vi "KlingerV2 OriginSearch.vi"(0 "VISA Rsrc":refnum<visa-resource-name>="SR530", 1 "UnitDem":u8(ring)=2 caption="Unités\nDemandées" items=["Pas", "mm", "ps"], 5 "Axe":u8(ring) items=["W", "X", "Y", "Z"], 7 "Moving Ref":refnum<vi>, 9 "Position Ref":refnum<vi>, 11 "error in":errorcluster, 12 "Set as Zero":bool) -> (2 "Pos Init":dbl caption="Position Initiale", 3 "Moving":bool caption="Déplacement\nen cours", 4 "PLimit":bool caption="Limite +", 6 "NLimit":bool caption="Limite -", 10 "Position":dbl format="%#.1f", 14 "Indcomm":string caption="Indicateur de commande", 15 "error out":errorcluster)   [LabVIEW 2019]
doc: "Ce VI envoie une commande de Mise à 0 au controlleur Klinger MC4. \n\nAxe : Sélectionner l'axe sur lequel effectuer la mise à zéro\n\nMoving Ref : Connecter une référence permet l'actualisation d'un afficheur de déplacement en cours en temp réelle\n\nPosition Ref: Connecter une référence permet l'actualisation d'un afficheur de position actuelle en temp réelle\n\nLimite + : Indique l'atteinte de l'interrupeur de fin de course positif\n\nLimite - : Indique l'atteinte de l'interrupeur de fin de course négatif\n\nPosition: Indique la position finale"
panel:
  out "Message D'erreur":string
  out "Erreur":bool
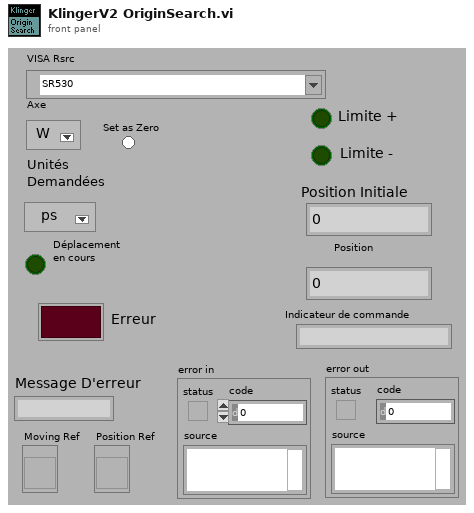
[diagram p1: front panel]
types:
  T1 = enum16{"Dem Pos Init", "Lire Pos Init", "Envoie Comm", "Dem Statut", "Lire Statut", "Attend RQS", "Erreur GPIB", "Dépl incomp", "Dépl comp"}
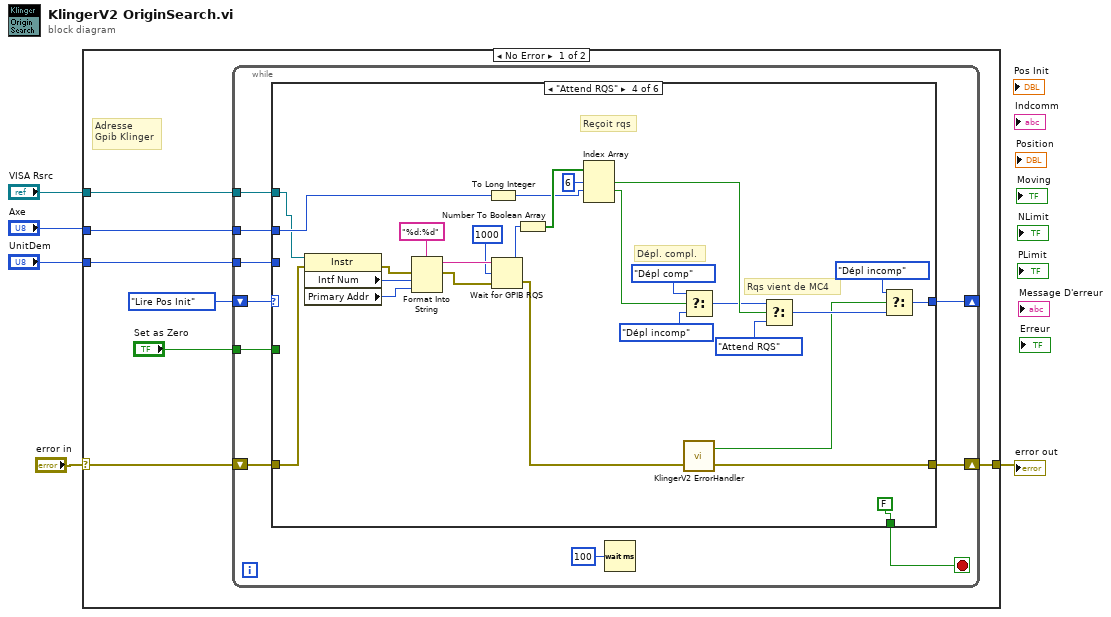
[diagram p0: block diagram]
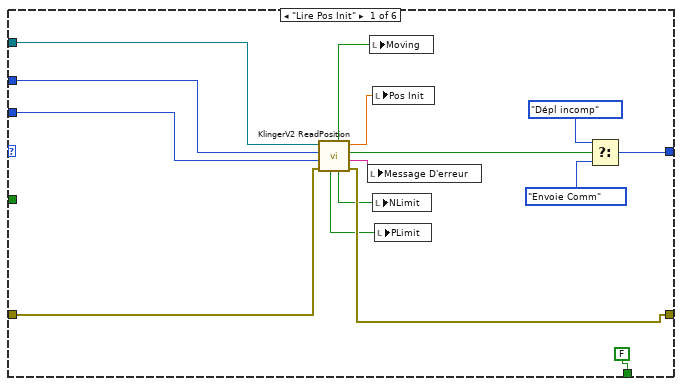
[diagram p2: hidden frame]
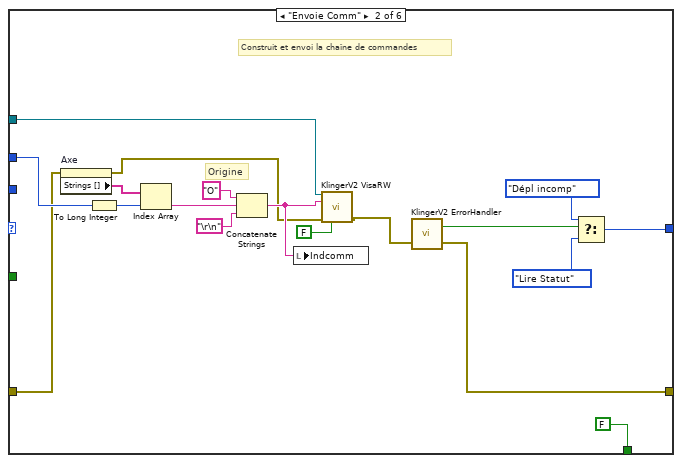
[diagram p3: hidden frame]
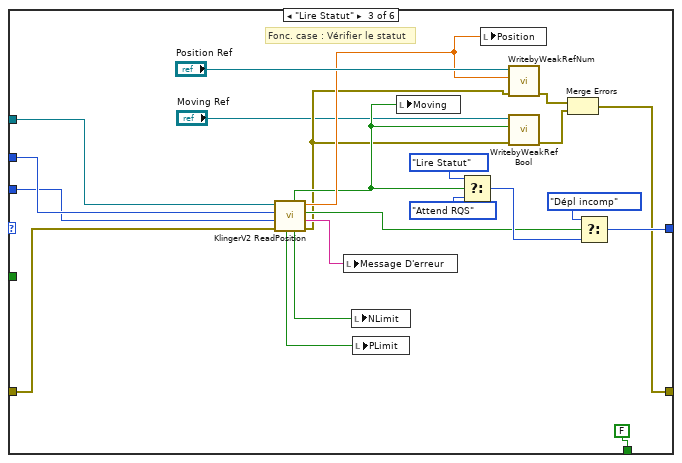
[diagram p4: hidden frame]
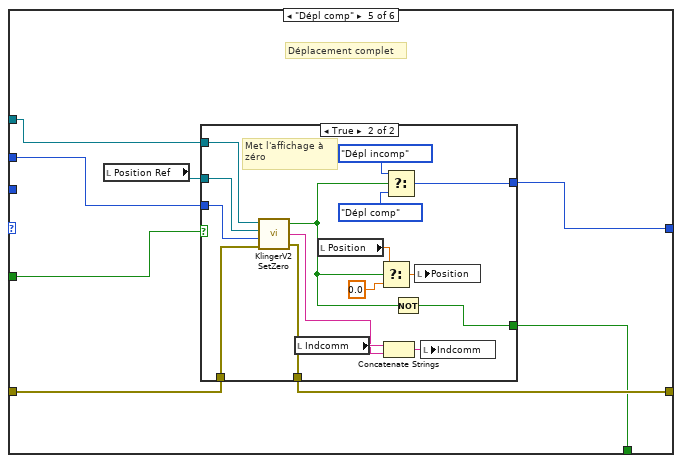
[diagram p5: hidden frame]
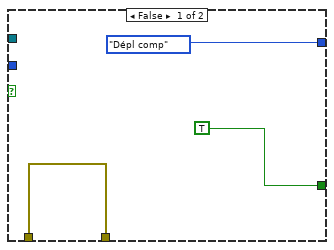
[diagram p6: hidden frame]
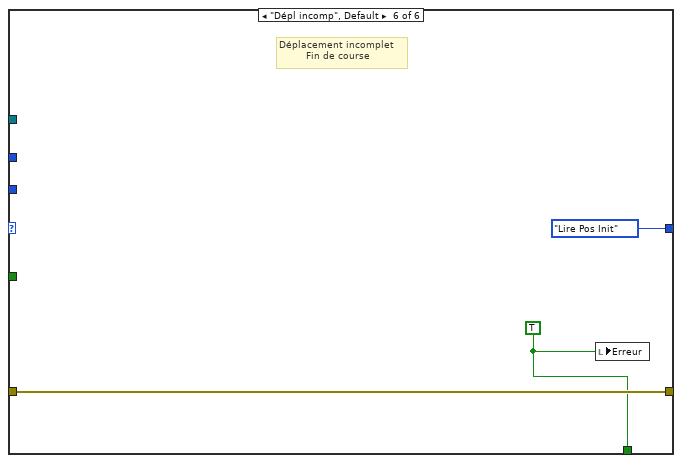
[diagram p7: hidden frame]
diagram:
  n1 = case shown="No Error" "error in" {
    selector: "error in" -> [w11 w135]
    tunnel: [w12 w135] -> w5
    tunnel: "VISA Rsrc" -> [w8 _]
    tunnel: "UnitDem" -> [w7 _]
    tunnel: "Axe" -> [w6 _]
    frame No Error {
      # "Adresse \nGpib Klinger"
      n2 = while {
        shift-right: [w21] -> w12
        shift-left: w11 -> [w20]
        tunnel: w6 -> [w19]
        shift-right: [w16] -> _
        shift-left: T1."Lire Pos Init" ("f") -> [w17]
        tunnel: "Set as Zero" -> [w15]
        tunnel: w7 -> [w14]
        tunnel: w8 -> [w13]
        stop <- w22 stop-if-true
        n3 = case shown="\"Attend RQS\"" w17 {
          tunnel: [FALSE FALSE FALSE FALSE w107 w132] -> w22
          tunnel: [w33 w45 w58 w90 w109 w133] -> w21
          tunnel: w20 -> [w31 w39 w71 w80 w110 w133]
          tunnel: w19 -> [w30 w52 w69 w104 w111 _]
          tunnel: [w34 w48 w74 w93 w108 T1."Lire Pos Init" ("f")] -> w16
          tunnel: w15 -> [_ _ _ _ w112 _]
          tunnel: w14 -> [w24 _ w65 _ _ _]
          tunnel: w13 -> [w23 w42 w64 w81 w105 _]
          frame "Lire Pos Init" {
            n4 = call <userlib>:"KlingerV2 ReadPosition.vi"("error in"=w31, "UnitDem"=w24, "Axe"=w30, "VISA Rsrc"=w23) -> ("error out"=w33:errorcluster, "Cont Error"=w25:string, "Statut"=w32:bool, "Position"=w29:dbl, "NLimit"=w27:bool, "Moving"=w28:bool, "PLimit"=w26:bool)  [unwired: 1 in]
            n5 = local write "Message D'erreur"(w25) -> ()
            n6 = local write "Moving"(w28) -> ()
            n7 = local write "Pos Init"(w29) -> ()
            n8 = local write "NLimit"(w27) -> ()
            n9 = local write "PLimit"(w26) -> ()
            n10 = Select(t=T1."Dépl incomp", s=w32, f=T1."Envoie Comm") -> (s? t:f=w34:T1)
          }
          frame "Envoie Comm" {
            # "Origine"
            # "Construit et envoi la chaîne de commandes"
            n11 = property on="Axe" class="MDér (strict)"(error in=w39) -> (error out=w38:errorcluster, "Strings []"=w55:string[])  [unwired: 1 in, 1 out]
            n12 = To Long Integer(number=w52) -> (32bit integer=w51:i32)
            n13 = Index Array(array=w55, index=w51) -> (element=w54:string)
            n14 = Concatenate Strings("O", w54, "\r\n") -> (w41:string)
            n15 = local write "Indcomm"(w41) -> ()
            n16 = call <userlib>:"KlingerV2 VisaRW.vi"("VISA Rsrc"=w42, "ChaineCom"=w41, "error in (no error)"=w38, "Lecture?(T)"=FALSE) -> ("error out"=w43:errorcluster)  [unwired: 7 in, 4 out]
            n17 = call <userlib>:"KlingerV2 ErrorHandler.vi"("error in (no error)"=w43) -> ("error out"=w45:errorcluster, "Erreur"=w44:bool)  [unwired: 1 in]
            n18 = Select(t=T1."Dépl incomp", s=w44, f=T1."Lire Statut") -> (s? t:f=w48:T1)
          }
          frame "Lire Statut" {
            # "Fonc. case : Vérifier le statut"
            n19 = call <userlib>:"KlingerV2 ReadPosition.vi"("error in"=w71, "UnitDem"=w65, "Axe"=w69, "VISA Rsrc"=w64) -> ("error out"=w60:errorcluster, "Cont Error"=w66:string, "Statut"=w70:bool, "Position"=w62:dbl, "NLimit"=w68:bool, "Moving"=w61:bool, "PLimit"=w67:bool)  [unwired: 1 in]
            n20 = local write "Message D'erreur"(w66) -> ()
            n21 = local write "NLimit"(w68) -> ()
            n22 = local write "PLimit"(w67) -> ()
            n23 = local write "Moving"(w61) -> ()
            n24 = Select(t=T1."Lire Statut", s=w61, f=T1."Attend RQS") -> (s? t:f=w72:T1)
            n25 = local write "Position"(w62) -> ()
            n26 = call <userlib>:"WritebyWeakRefNum.vi"("error in"=w60, "Valeur"=w62, "Control Ref"="Position Ref") -> ("error out"=w59:errorcluster)  [unwired: 8 in]
            n27 = call <userlib>:"WritebyWeakRefBool.vi"("error in"=w60, "Valeur"=w61, "Control Ref"="Moving Ref") -> ("error out"=w56:errorcluster)  [unwired: 8 in]
            n28 = Merge Errors(w59, w56) -> (w58:errorcluster)
            n29 = Select(t=T1."Dépl incomp", s=w70, f=w72) -> (s? t:f=w74:T1)
          }
          frame "Attend RQS" {
            # "Dépl. compl."
            # "Rqs vient de MC4"
            # "Reçoit rqs"
            n30 = property class="Instr"(reference=w81, error in=w80) -> (error out=w85:errorcluster, "Intf Num"=w83:u16, "Primary Addr"=w84:u16)  [unwired: 1 out]
            n31 = Format Into String(format string="%d:%d" ("chaîne de format"), error in=w85, w83, w84) -> (resulting string=w86:string, error out=w87:errorcluster)  [unwired: 1 in]
            n32 = To Long Integer(number=w104) -> (32bit integer=w99:i32)
            n33 = Wait for GPIB RQS(2:w87, 3:1000 ("timeout (25000 ms)"), 4:w86) -> (0:w79:errorcluster, 1:w78:i16)
            n34 = Number To Boolean Array(number=w78) -> (Boolean array=w103:bool[])
            n35 = Index Array(array=w103, index #1=6 ("index"), index #2=w99) -> (element #1=w101:bool, element #2=w98:bool)  [unwired: 1 in, 1 out]
            n36 = Select(t=T1."Dépl comp", s=w98, f=T1."Dépl incomp") -> (s? t:f=w97:T1)
            n37 = call <userlib>:"KlingerV2 ErrorHandler.vi"("error in (no error)"=w79) -> ("error out"=w90:errorcluster, "Erreur"=w89:bool)  [unwired: 1 in]
            n38 = Select(t=w97, s=w101, f=T1."Attend RQS") -> (s? t:f=w92:T1)
            n39 = Select(t=T1."Dépl incomp", s=w89, f=w92) -> (s? t:f=w93:T1)
          }
          frame "Dépl comp" {
            # "Déplacement complet"
            n40 = local read "Position Ref"() -> (w106:refnum<vi>)
            n41 = case shown="True" w112 {
              tunnel: w111 -> [_ w125]
              tunnel: w110 -> [w115 w126]
              tunnel: [w115 w127] -> w109
              tunnel: [T1."Dépl comp" w129] -> w108
              tunnel: [TRUE ("Stop") w128] -> w107
              tunnel: w106 -> [_ w117]
              tunnel: w105 -> [_ w116]
              frame False {
              }
              frame True {
                # "Met l'affichage à \nzéro"
                n42 = call <userlib>:"KlingerV2 SetZero.vi"("VISA Rsrc"=w116, "Position Ref"=w117, "Axe"=w125, "error in"=w126) -> ("Statut"=w124:bool, "Ind Comm"=w118:string, "error out"=w127:errorcluster)  [unwired: 1 in]
                n43 = local read "Indcomm"() -> (w120:string)
                n44 = local read "Position"() -> (w122:dbl)
                n45 = Select(t=w122, s=w124, f=0.0) -> (s? t:f=w123:dbl)
                n46 = Concatenate Strings(w120, w118) -> (w119:string)
                n47 = Select(t=T1."Dépl incomp", s=w124, f=T1."Dépl comp") -> (s? t:f=w129:T1)
                n48 = Not(x=w124) -> (.not. x?=w128:bool)
                n49 = local write "Position"(w123) -> ()
                n50 = local write "Indcomm"(w119) -> ()
              }
            }
          }
          frame "Dépl incomp", Default {
            w132 = TRUE ("Stop")
            # "Déplacement incomplet\n         Fin de course"
            n51 = local write "Erreur"(w132) -> ()
          }
        }
        n52 = Wait (ms)(milliseconds to wait=u32 100) -> ()  [unwired: 1 out]
      }
    }
    frame Error {
    }
  }
  "error out" <- w5
